vi "Test wykresow.vi"() -> ()   [LabVIEW 2014]
uses:
  <vilib>/Utility/miscctls.llb/LVPositionTypeDef.ctl
panel:
  out "Width+Left":u32
  out "Bounds:Area Width":u32
  out "Position:Left 2":i32
  out "Legend:Position":T1
  out "Array":string[](array[string])
  out "Position:Left":i32
  out "Plot Area:Size:Width":u32
  in  "skale":bool
  in  "stop":bool
  in  "Skale 2":bool[](array[boolean])
  out "Waveform 2":dbl[](graph)
  in  "Skale 1":bool[](array[boolean])
  in  "niewidoczna":bool
  out "Y Scale.Grid Colors:Minor Color":u32
  out "Y Scale.Grid Colors:Major Color":u32
  out "X Scale.Grid Colors:Minor Color":u32
  out "X Scale.Grid Colors:Major Color":u32
  out "Waveform 1":dbl[](graph)
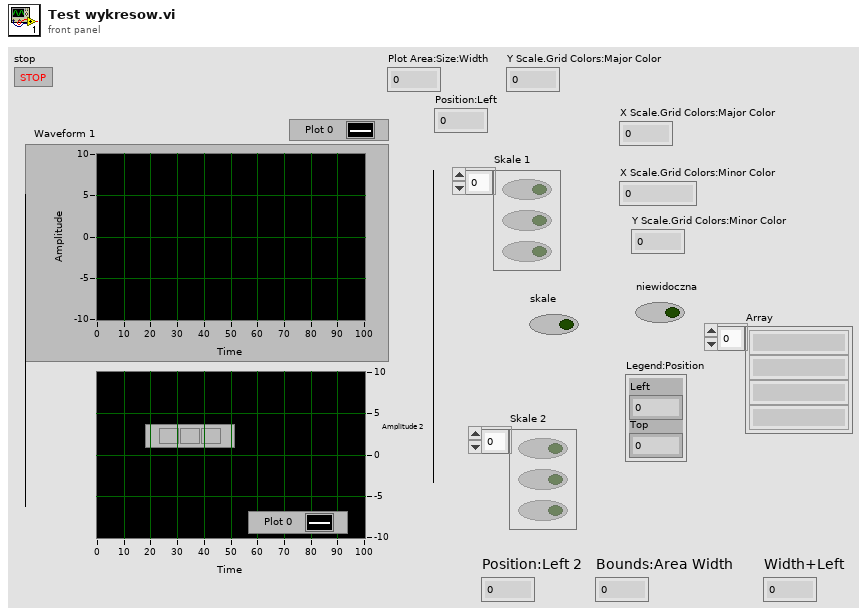
[diagram p1: front panel]
types:
  T1 = typedef "LVPositionTypeDef.ctl" = cluster{"Left":i32, "Top":i32}
  T2 = typedef "LVRectTypeDef.ctl" = cluster{"Left":i16, "Top":i16, "Right":i16, "Bottom":i16}
  T3 = typedef "LVPoint32TypeDef.ctl" = cluster{"Horizontal":i32, "Vertical":i32}
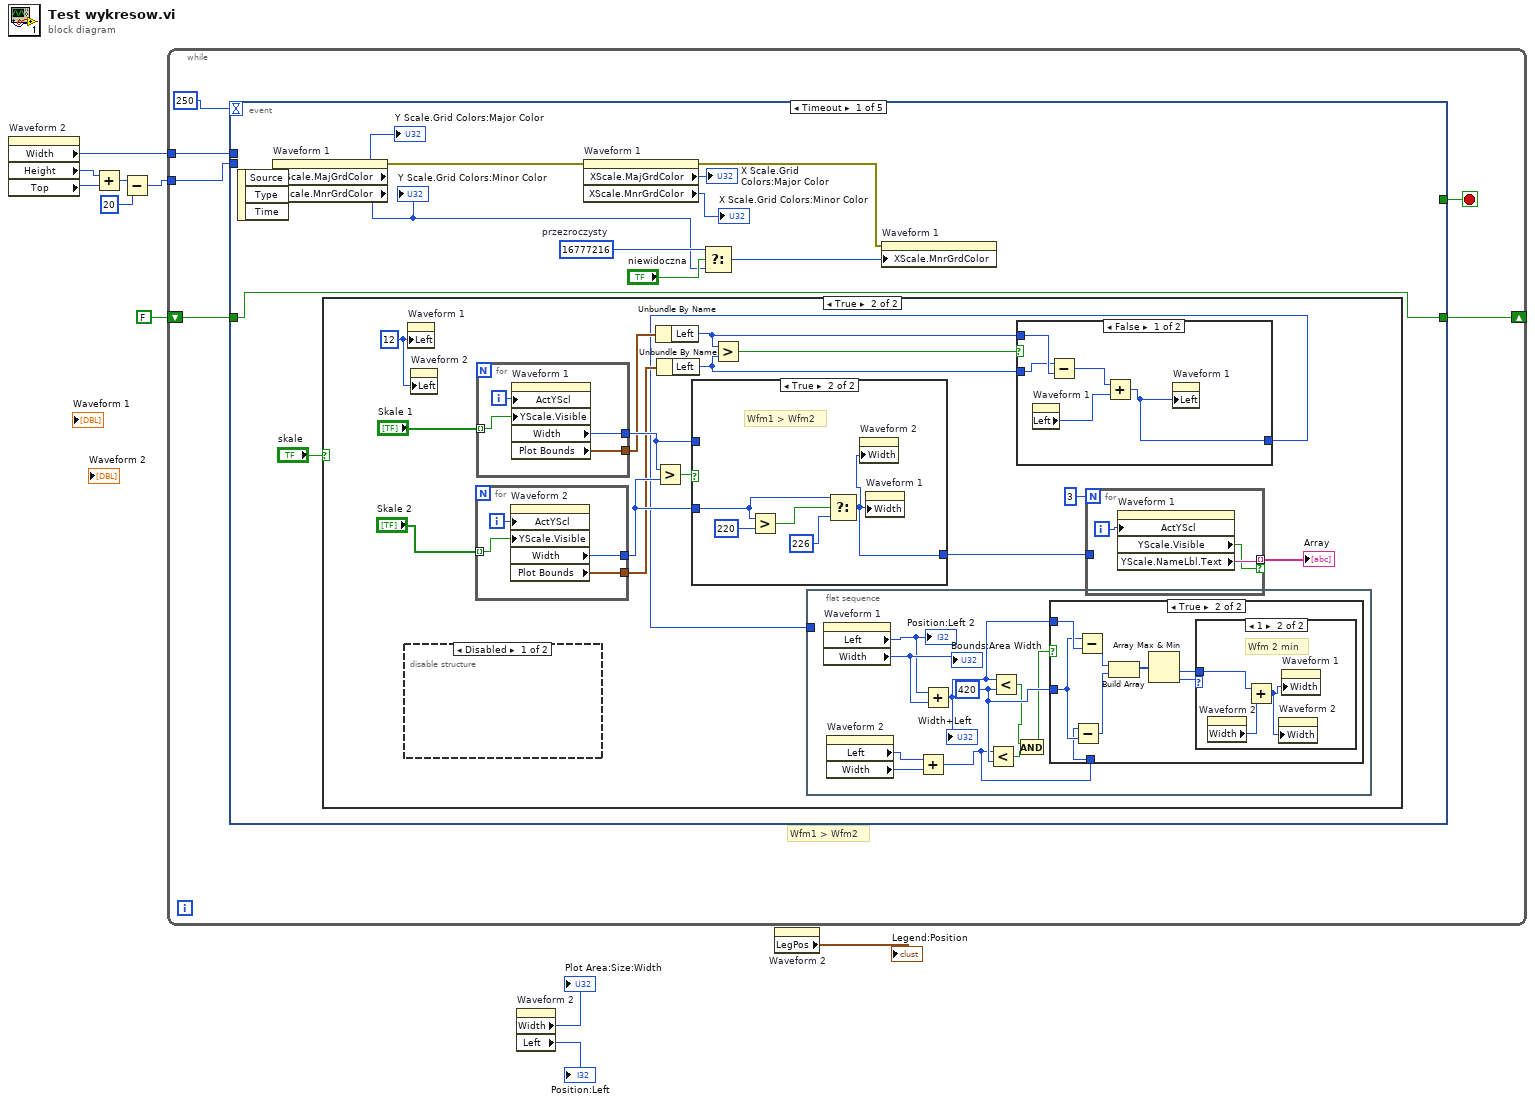
[diagram p0: block diagram]
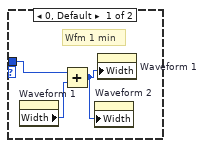
[diagram p5: hidden frame]
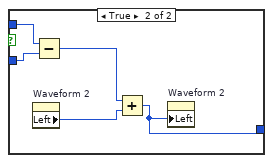
[diagram p6: hidden frame]
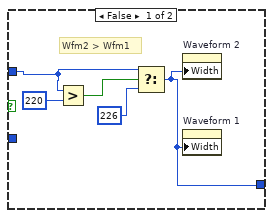
[diagram p7: hidden frame]
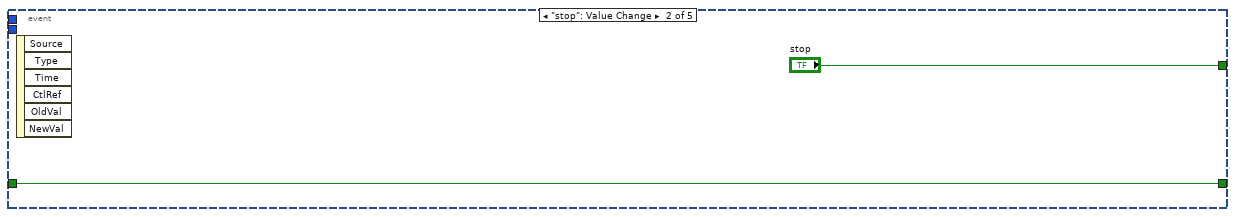
[diagram p8: hidden frame]
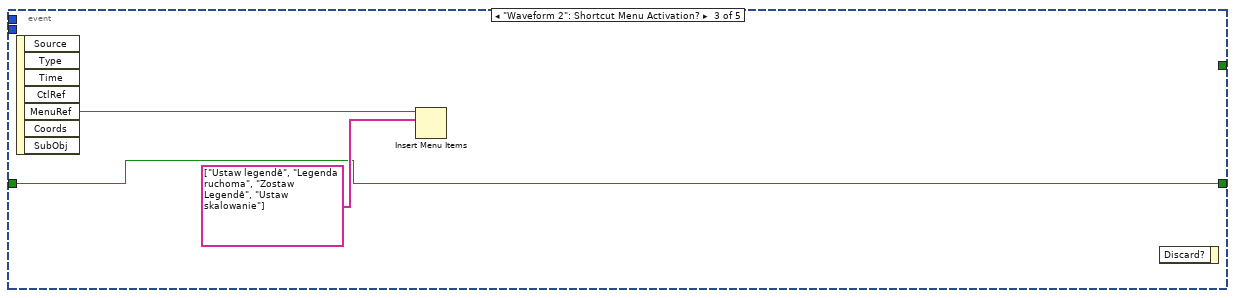
[diagram p9: hidden frame]
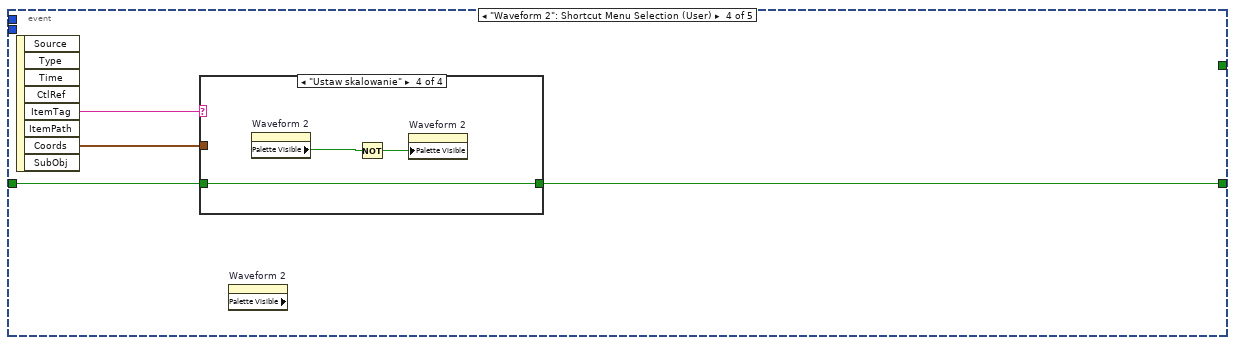
[diagram p10: hidden frame]
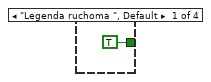
[diagram p11: hidden frame]
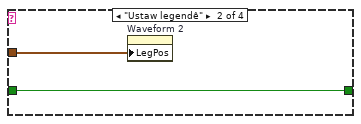
[diagram p12: hidden frame]
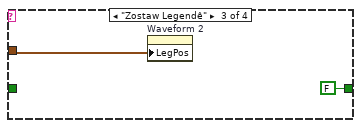
[diagram p13: hidden frame]
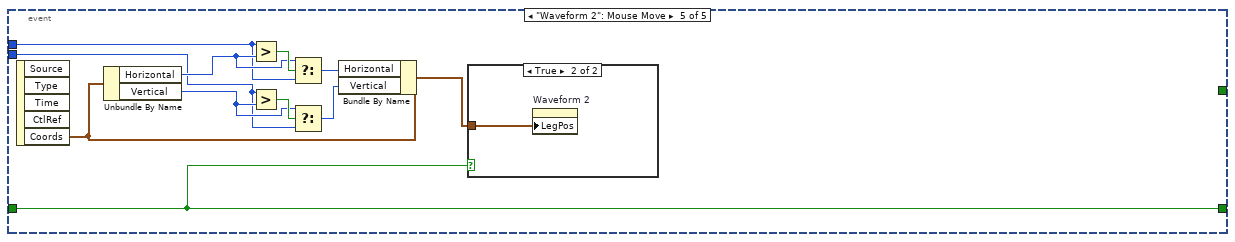
[diagram p14: hidden frame]
diagram:
  n1 = property on="Waveform 2" class="WFGraph (strict)"() -> ("Width"=w6:u32, "Height"=w5:u32, "Top"=w4:i32)  [unwired: 2 in, 2 out]
  n2 = Add(x=w5, y=w4) -> (x+y=w2:u32)
  n3 = Subtract(x=w2, y=u32 20) -> (x-y=w3:u32)
  n4 = while {
    shift-right: [w13] -> _
    shift-left: FALSE -> [w14]
    tunnel: w6 -> [w12]
    tunnel: w3 -> [w11]
    stop <- w15 stop-if-true
    # "Wfm1 > Wfm2"
    n5 = event shown="[0] Timeout" {
      selector: _ -> [_ _ _ _ _]
      dyn-events: _ -> [_ _ _ _ _]
      timeout: 250 -> [_ _ _ _ _]
      tunnel: [_ "stop" _ _ _] -> w15
      tunnel: w14 -> [w17 w98 w100 w104 w125]
      tunnel: [w17 w98 w100 w103 w125] -> w13
      tunnel: w12 -> [_ _ _ _ w121]
      tunnel: w11 -> [_ _ _ _ w115]
      event Timeout {
        w20 = u32 16777216  # przezroczysty
        n6 = event-data() -> ()  [unwired: 1 in, 3 out]
        n7 = property on="Waveform 1" class="WFGraph (strict)"() -> (error out=w25:errorcluster, "YScale.MajGrdColor"=→"Y Scale.Grid Colors:Major Color":u32, "YScale.MnrGrdColor"=w19:u32)  [unwired: 2 in, 1 out]
        "Y Scale.Grid Colors:Minor Color" <- w19
        n8 = case shown="True" "skale" {
          frame False {
          }
          frame True {
            w32 = 12 ("Position:Left")
            n9 = disable-structure shown="Disabled" {
              frame Disabled {
              }
              frame Enabled {
              }
            }
            n10 = property on="Waveform 1" class="WFGraph (strict)"("Left"=w32) -> ()  [unwired: 2 in, 2 out]
            n11 = property on="Waveform 2" class="WFGraph (strict)"("Left"=w32) -> ()  [unwired: 2 in, 2 out]
            n12 = for {
              tunnel: "Skale 2" -> [w92] mode=indexing
              tunnel: [w91] -> w39
              tunnel: [w90] -> w37
              i -> [w93]
              n13 = property on="Waveform 2" class="WFGraph (strict)"("ActYScl"=w93, "YScale.Visible"=w92) -> ("Width"=w91:u32, "Plot Bounds"=w90:T2)  [unwired: 2 in, 2 out]
            }
            n14 = for {
              tunnel: "Skale 1" -> [w96] mode=indexing
              tunnel: [w95] -> w38
              tunnel: [w94] -> w36
              i -> [w97]
              n15 = property on="Waveform 1" class="WFGraph (strict)"("ActYScl"=w97, "YScale.Visible"=w96) -> ("Width"=w95:u32, "Plot Bounds"=w94:T2)  [unwired: 2 in, 2 out]
            }
            n16 = Greater?(x=w38, y=w39) -> (0:w40:bool)
            n17 = Unbundle By Name(w36) -> ("Left"=w34:i16)
            n18 = Unbundle By Name(w37) -> ("Left"=w33:i16)
            n19 = case shown="True" w40 {
              tunnel: w39 -> [_ w87]
              tunnel: w38 -> [w81 _]
              tunnel: [w80 w85] -> w30
              frame False {
                # "Wfm2 > Wfm1"
                n20 = Greater?(x=w81, y=u32 220) -> (0:w83:bool)
                n21 = Select(t=w81, s=w83, f=u32 226) -> (s? t:f=w80:u32)
                n22 = property on="Waveform 2" class="WFGraph (strict)"("Width"=w80) -> ()  [unwired: 2 in, 2 out]
                n23 = property on="Waveform 1" class="WFGraph (strict)"("Width"=w80) -> ()  [unwired: 2 in, 2 out]
              }
              frame True {
                # "Wfm1 > Wfm2"
                n24 = Greater?(x=w87, y=u32 220) -> (0:w88:bool)
                n25 = Select(t=w87, s=w88, f=u32 226) -> (s? t:f=w85:u32)
                n26 = property on="Waveform 2" class="WFGraph (strict)"("Width"=w85) -> ()  [unwired: 2 in, 2 out]
                n27 = property on="Waveform 1" class="WFGraph (strict)"("Width"=w85) -> ()  [unwired: 2 in, 2 out]
              }
            }
            n28 = Greater?(x=w34, y=w33) -> (0:w35:bool)
            n29 = flat-sequence {
              tunnel: w28 -> [_]
              frame #0 {
                w47 = u32 420 ("y")
                n30 = property on="Waveform 1" class="WFGraph (strict)"() -> ("Left"=w51:i32, "Width"=w52:u32)  [unwired: 2 in, 2 out]
                "Position:Left 2" <- w51
                "Bounds:Area Width" <- w52
                n31 = property on="Waveform 2" class="WFGraph (strict)"() -> ("Left"=w49:i32, "Width"=w48:u32)  [unwired: 2 in, 2 out]
                n32 = Add(x=w49, y=w48) -> (x+y=w43:u32)
                n33 = Add(x=w51, y=w52) -> (x+y=w50:u32)
                "Width+Left" <- w50
                n34 = Less?(x=w43, y=w47) -> (x < y?=w46:bool)
                n35 = Less?(x=w50, y=w47) -> (x < y?=w45:bool)
                n36 = And(x=w45, y=w46) -> (x .and. y?=w44:bool)
                n37 = case shown="True" w44 {
                  tunnel: w50 -> [_ w60]
                  tunnel: w47 -> [_ w59]
                  tunnel: w43 -> [_ w58]
                  frame False {
                  }
                  frame True {
                    n38 = Subtract(x=w58, y=w59) -> (x-y=w56:u32)
                    n39 = Subtract(x=w59, y=w60) -> (x-y=w57:u32)
                    n40 = Build Array(w57, w56) -> (w55:u32[])
                    n41 = Array Max & Min(array=w55) -> (min value=w53:u32, min index (indices)=w54:i32)  [unwired: 2 out]
                    n42 = case shown="1" w54 {
                      tunnel: w53 -> [w61 w65]
                      frame 0, Default {
                        # "Wfm 1 min"
                        n43 = property on="Waveform 1" class="WFGraph (strict)"() -> ("Width"=w63:u32)  [unwired: 2 in, 2 out]
                        n44 = Add(x=w61, y=w63) -> (x+y=w62:u32)
                        n45 = property on="Waveform 2" class="WFGraph (strict)"("Width"=w62) -> ()  [unwired: 2 in, 2 out]
                        n46 = property on="Waveform 1" class="WFGraph (strict)"("Width"=w62) -> ()  [unwired: 2 in, 2 out]
                      }
                      frame 1 {
                        # "Wfm 2 min"
                        n47 = property on="Waveform 2" class="WFGraph (strict)"() -> ("Width"=w64:u32)  [unwired: 2 in, 2 out]
                        n48 = Add(x=w65, y=w64) -> (x+y=w66:u32)
                        n49 = property on="Waveform 2" class="WFGraph (strict)"("Width"=w66) -> ()  [unwired: 2 in, 2 out]
                        n50 = property on="Waveform 1" class="WFGraph (strict)"("Width"=w66) -> ()  [unwired: 2 in, 2 out]
                      }
                    }
                  }
                }
              }
            }
            n51 = case shown="False" w35 {
              tunnel: w34 -> [w73 w79]
              tunnel: w33 -> [w72 w78]
              tunnel: [w70 w75] -> w28
              frame False {
                n52 = property on="Waveform 1" class="WFGraph (strict)"() -> ("Left"=w71:i32)  [unwired: 2 in, 2 out]
                n53 = Subtract(x=w72, y=w73) -> (x-y=w74:i16)
                n54 = Add(x=w74, y=w71) -> (x+y=w70:i32)
                n55 = property on="Waveform 1" class="WFGraph (strict)"("Left"=w70) -> ()  [unwired: 2 in, 2 out]
              }
              frame True {
                n56 = property on="Waveform 2" class="WFGraph (strict)"() -> ("Left"=w77:i32)  [unwired: 2 in, 2 out]
                n57 = Subtract(x=w79, y=w78) -> (x-y=w76:i16)
                n58 = Add(x=w76, y=w77) -> (x+y=w75:i32)
                n59 = property on="Waveform 2" class="WFGraph (strict)"("Left"=w75) -> ()  [unwired: 2 in, 2 out]
              }
            }
            n60 = for {
              N: 3 -> [_]
              tunnel: w30 -> [_]
              tunnel: [w68] -> w29 mode=indexing if=w67
              i -> [w69]
              n61 = property on="Waveform 1" class="WFGraph (strict)"("ActYScl"=w69) -> ("YScale.Visible"=w67:bool, "YScale.NameLbl.Text"=w68:string)  [unwired: 2 in, 2 out]
            }
            "Array" <- w29
          }
        }
        n62 = property on="Waveform 1" class="WFGraph (strict)"(error in=w25) -> (error out=w24:errorcluster, "XScale.MajGrdColor"=→"X Scale.Grid Colors:Major Color":u32, "XScale.MnrGrdColor"=→"X Scale.Grid Colors:Minor Color":u32)  [unwired: 1 in, 1 out]
        n63 = Select(t=w20, s="niewidoczna", f=w19) -> (s? t:f=w27:u32)
        n64 = property on="Waveform 1" class="WFGraph (strict)"(error in=w24, "XScale.MnrGrdColor"=w27) -> ()  [unwired: 1 in, 2 out]
      }
      event "stop": Value Change {
        n65 = event-data() -> ()  [unwired: 1 in, 6 out]
      }
      event "Waveform 2": Shortcut Menu Activation? {
        n66 = event-data() -> ("MenuRef"=w102:refnum<k9>)  [unwired: 1 in, 6 out]
        n67 = Insert Menu Items(8:string[] ["Ustaw legendê", "Legenda ruchoma", "Zostaw Legendê", "Ustaw skalowanie"] ("item names"), 9:w102) -> ()  [unwired: 4 in, 3 out]
        n68 = event-data() -> ()  [unwired: 2 in, 1 out]
      }
      event "Waveform 2": Shortcut Menu Selection (User) {
        n69 = event-data() -> ("ItemTag"=w105:string, "Coords"=w106:T3)  [unwired: 1 in, 6 out]
        n70 = case shown="\"Ustaw skalowanie\"" w105 {
          tunnel: w106 -> [_ w109 w110 _]
          tunnel: w104 -> [_ w108 _ w114]
          tunnel: [TRUE w108 FALSE w114] -> w103
          frame "Legenda ruchoma ", Default {
          }
          frame "Ustaw legendê" {
            n71 = property on="Waveform 2" class="WFGraph (strict)"("LegPos"=w109) -> ()  [unwired: 2 in, 2 out]
          }
          frame "Zostaw Legendê" {
            n72 = property on="Waveform 2" class="WFGraph (strict)"("LegPos"=w110) -> ()  [unwired: 2 in, 2 out]
          }
          frame "Ustaw skalowanie" {
            n73 = property on="Waveform 2" class="WFGraph (strict)"() -> ("Palette Visible"=w112:bool)  [unwired: 2 in, 2 out]
            n74 = Not(x=w112) -> (.not. x?=w113:bool)
            n75 = property on="Waveform 2" class="WFGraph (strict)"("Palette Visible"=w113) -> ()  [unwired: 2 in, 2 out]
          }
        }
        n76 = property on="Waveform 2" class="WFGraph (strict)" props=["Palette Visible"]() -> ()  [unwired: 2 in, 3 out]
      }
      event "Waveform 2": Mouse Move {
        n77 = event-data() -> ("Coords"=w119:T3)  [unwired: 1 in, 4 out]
        n78 = Unbundle By Name(w119) -> ("Horizontal"=w122:i32, "Vertical"=w116:i32)
        n79 = Greater?(x=w121, y=w122) -> (0:w123:bool)
        n80 = Greater?(x=w115, y=w116) -> (0:w118:bool)
        n81 = Select(t=w122, s=w123, f=w121) -> (s? t:f=w120:u32)
        n82 = Select(t=w116, s=w118, f=w115) -> (s? t:f=w117:u32)
        n83 = Bundle By Name(cluster=w119, "Horizontal"=w120, "Vertical"=w117) -> (w124:T3)
        n84 = case shown="True" w125 {
          tunnel: w124 -> [_ w126]
          frame False {
          }
          frame True {
            n85 = property on="Waveform 2" class="WFGraph (strict)"("LegPos"=w126) -> ()  [unwired: 2 in, 2 out]
          }
        }
      }
    }
  }
  n86 = property on="Waveform 2" class="WFGraph (strict)"() -> ("Width"=→"Plot Area:Size:Width":u32, "Left"=→"Position:Left":i32)  [unwired: 2 in, 2 out]
  n87 = property on="Waveform 2" class="WFGraph (strict)"() -> ("LegPos"=→"Legend:Position":T1)  [unwired: 2 in, 2 out]
